vi "PathPlanner_Cmd_Follow_Internal_TriggerEvents.vi"(8 "TrigerEvents":bool, 9 "Reset":bool, 10 "TrajectoryTimeStampSecs":dbl, 11 "PathPlannerTrajectoryEvents":T1) -> ()   [LabVIEW 2019, in "PathPlanner24.lvlib"]
doc: "This is an internal function. It is not to be called by end users."
uses:
  PathPlanner24.lvlib
  TypeDef/PathPlannerTrajectoryEvents.ctl
  TypeDef/PathPlannerTrajectoryEvent.ctl
  TypeDef/PathPlannerCommandUtil.ctl
  ENum/PathPlanner_CommandUtilType_ENUM.ctl
  <vilib>/Utility/error.llb/Clear Errors.vi
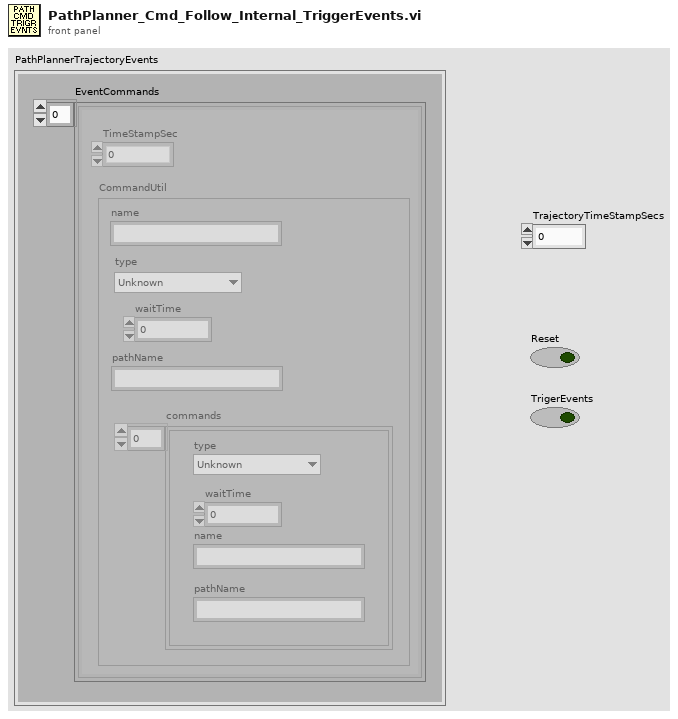
[diagram p1: front panel]
types:
  T1 = typedef "PathPlanner24.lvlib/PathPlannerTrajectoryEvents.ctl" = cluster{"EventCommands":T2[]}
  T2 = typedef "PathPlanner24.lvlib/PathPlannerTrajectoryEvent.ctl" = cluster{"TimeStampSec":dbl, "CommandUtil":T3}
  T3 = typedef "PathPlanner24.lvlib/PathPlannerCommandUtil.ctl" = cluster{"waitTime":dbl, "name":string, "pathName":string, "commands":cluster{"type":T4, "waitTime":dbl, "name":string, "pathName":string}[], "type":T4}
  T4 = typedef "PathPlanner24.lvlib/PathPlanner_CommandUtilType_ENUM.ctl" = enum16{"Unknown", "Wait", "Named", "Path", "Sequential", "Parallel", "Race", "Deadline"}
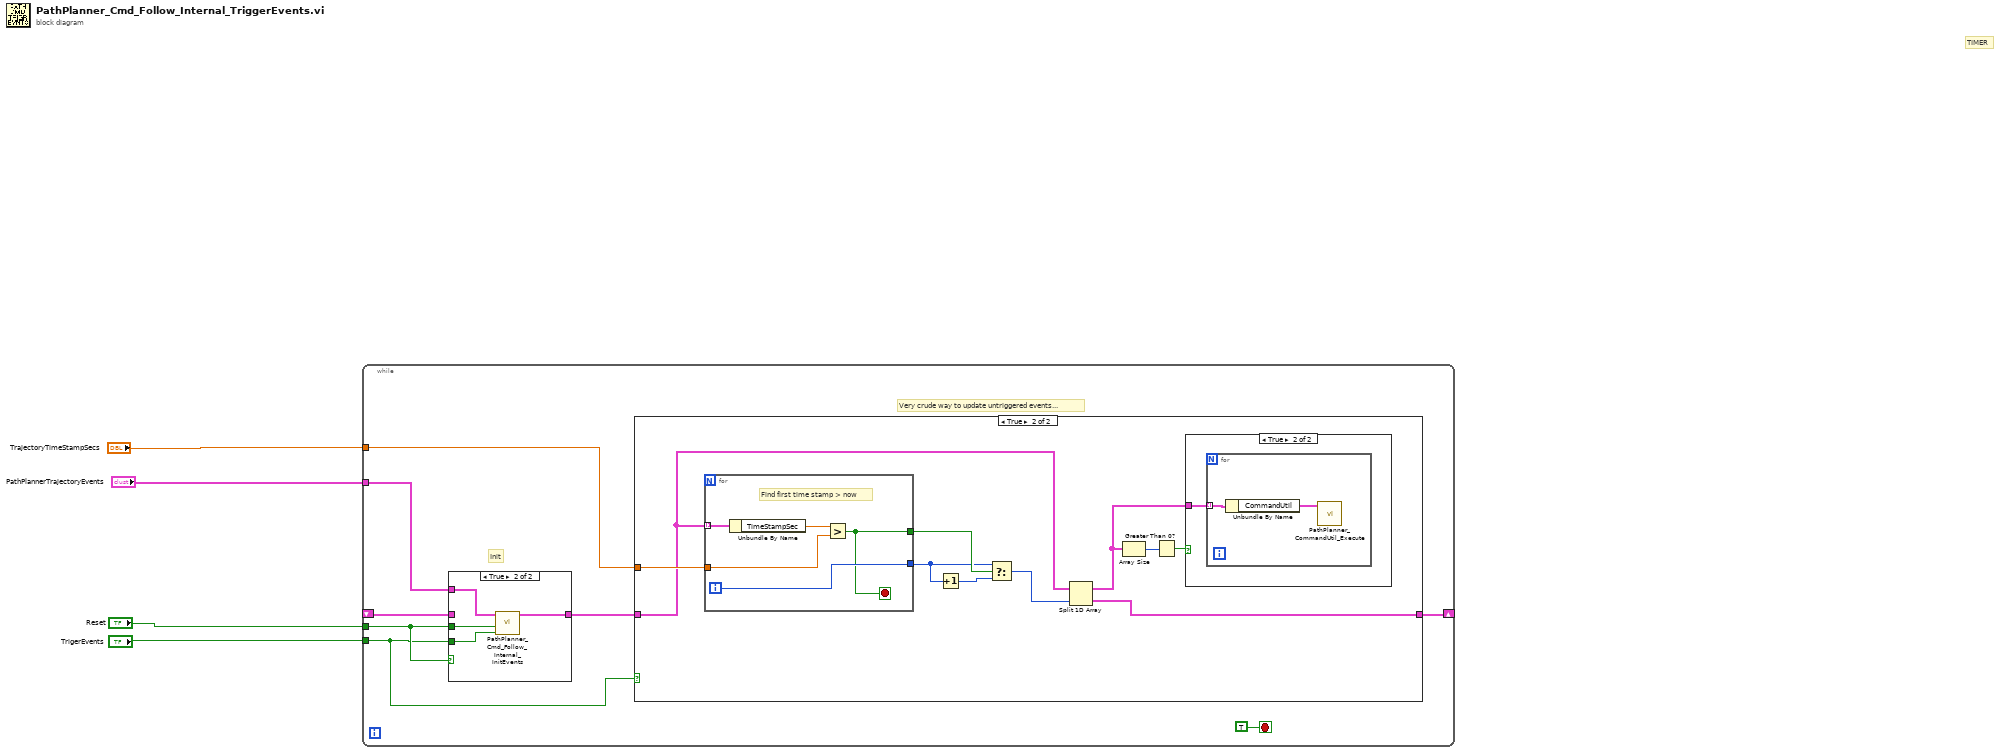
[diagram p0: block diagram]
diagram:
  # "TIMER"
  n1 = while {
    tunnel: "Reset" -> [w11]
    tunnel: "TrigerEvents" -> [w8]
    tunnel: "PathPlannerTrajectoryEvents" -> [w10]
    shift-right: [w5] -> _
    shift-left: _ -> [w9]
    tunnel: "TrajectoryTimeStampSecs" -> [w6]
    stop <- TRUE stop-if-true
    # "Very crude way to update untriggered events..."
    # "Init"
    n2 = case shown="True" w11 {
      tunnel: w8 -> [_ w36]
      tunnel: w11 -> [_ w35]
      tunnel: w10 -> [_ w34]
      tunnel: [w32 w33] -> w7
      tunnel: w9 -> [w32 _]
      frame False {
      }
      frame True {
        n3 = call "PathPlanner_Cmd_Follow_Internal_InitEvents.vi"("TrigerEvents"=w36, "Reset In"=w35, "TrajectoryEventCommands"=w34) -> ("UntriggeredEvents"=w33:T2[])  [unwired: 8 in]
      }
    }
    n4 = case shown="True" w8 {
      tunnel: w7 -> [w13 w22]
      tunnel: w6 -> [_ w23]
      tunnel: [w13 w21] -> w5
      frame False {
      }
      frame True {
        n5 = for {
          tunnel: w22 -> [w31] mode=indexing
          tunnel: w23 -> [w29]
          tunnel: [w28] -> w15
          tunnel: [w27] -> w17
          i -> [w28]
          stop <- w27 stop-if-true
          # "Find first time stamp > now"
          n6 = Unbundle By Name(w31) -> ("TimeStampSec"=w30:dbl)
          n7 = Greater?(x=w30, y=w29) -> (0:w27:bool)
        }
        n8 = Increment(x=w15) -> (x+1=w14:i32)
        n9 = Select(t=w15, s=w17, f=w14) -> (s? t:f=w16:i32)
        n10 = Split 1D Array(array=w22, index=w16) -> (first subarray=w20:T2[], second subarray=w21:T2[])
        n11 = Array Size(array=w20) -> (size(s)=w19:i32)
        n12 = Greater Than 0?(x=w19) -> (x > 0?=w18:bool)
        n13 = case shown="True" w18 {
          tunnel: w20 -> [_ w24]
          frame False {
          }
          frame True {
            n14 = for {
              tunnel: w24 -> [w26] mode=indexing
              n15 = Unbundle By Name(w26) -> ("CommandUtil"=w25:T3)
              n16 = call "PathPlanner_CommandUtil_Execute.vi"("Command"=w25) -> ()  [unwired: 11 in]
            }
          }
        }
      }
    }
  }
